vi "Channel Data to FP Cluster.vi"(0 "CS++DCPwrChannelData in":refnum<class "CS++DCPwrChannelData.lvclass">, 5 "Channel Index":i32, 11 "Error In":errorcluster) -> (2 "Maximum Limits":T2 {"Max Voltage Level" format="%^.3g"; "Max Current Limit" format="%^.3g"}, 3 "Range":cluster{"Range Type":i32, "Range":dbl}={"Range Type"=1, "Range"=0.0} {"Range" format="%^.3g"; "Range Type" items=["Voltage"=1, "Current"=0]}, 4 "CS++DCPwrChannelData out":refnum<class "CS++DCPwrChannelData.lvclass">, 6 "Output Enable":bool caption="Channel Enabled", 8 "Output State":i32(ring) items=["Constant Voltage"=0, "Constant Current"=1, "Unregulated"=4, "Over Voltage"=2, "Over Current"=3], 10 "Current":T1 {"Behavior" items=["Regulate", "Trip"]; "Current Limit" format="%^.3g"}, 13 "Trigger":T4 {"Triggered I-Limit" format="%^.6g"; "Triggered U-Level" format="%^.6g"; "Trigger Source" items=["Immediate", "External", "Software", "TTL0", "TTL1", "TTL2", "TTL3", "TTL4", "TTL5", "TTL6", "TTL7", "ECL0", "ECL1", "PXI Star", "RTSI 0", "RTSI 1", "RTSI 2", "RTSI 3", "RTSI 4", "RTSI 5", "RTSI 6"]}, 14 "OVP":T3 {"OVP Limit" format="%^.3g"}, 15 "Error Out":errorcluster)   [LabVIEW 2015, in "CS++DCPwrGui.lvlib" / "CS++DCPwrChannelData.lvclass"]
doc: "Return channel data in cluster ."
uses:
  CS++DCPwrChannelData/CS++DCPwrChannelData.lvclass
  CS++DCPwrChannelData/CS++DCPwrChannelData.lvclass/CS++DCPwrChannelData.ctl
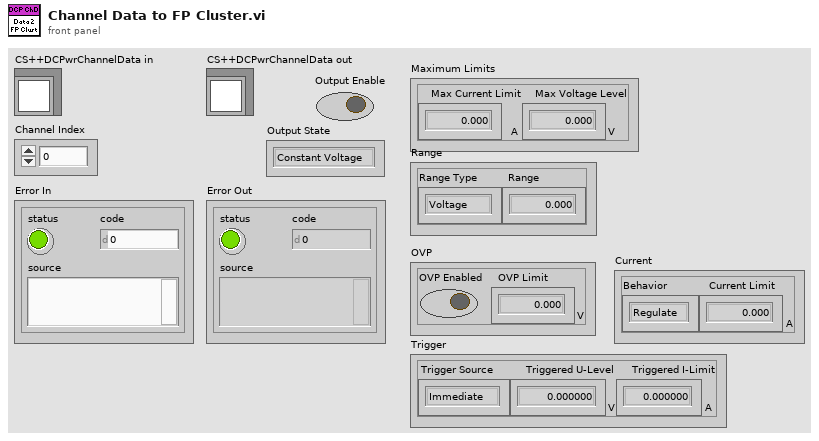
[diagram p1: front panel]
types:
  T1 = cluster{"Behavior":i32, "Current Limit":dbl[unit]}
  T2 = cluster{"Max Current Limit":dbl[unit], "Max Voltage Level":dbl[unit]}
  T3 = cluster{"OVP Enabled":bool, "OVP Limit":dbl[unit]}
  T4 = cluster{"Trigger Source":i32, "Triggered U-Level":dbl[unit], "Triggered I-Limit":dbl[unit]}
  T5 = cluster{"max current limit":dbl[unit], "max voltage level":dbl[unit]}
  T6 = cluster{"range type (Voltage)":i32, "range (0.0)":dbl}
  T7 = cluster{"behavior (regulate)":i32, "limit (0.0 Amps)":dbl[unit]}
  T8 = cluster{"enabled (true)":bool, "limit (0.0 Volts)":dbl[unit]}
  T9 = cluster{"source (Immediate)":i32, "triggered level (0.0 Volts)":dbl[unit], "triggered limit (0.0 Amps)":dbl[unit]}
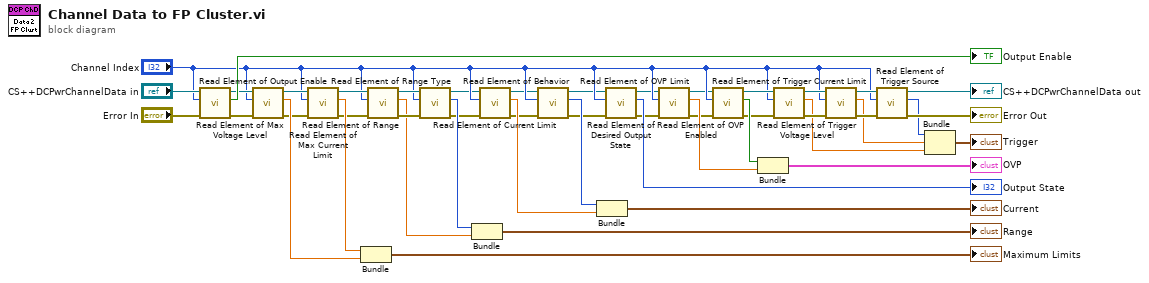
[diagram p0: block diagram]
diagram:
  n1 = call "Read Element of Output Enable.vi"("error in (no error)"="Error In", "index"="Channel Index", "CS++DCPwrChannelData in"="CS++DCPwrChannelData in") -> ("error out"=w41:errorcluster, "enabled (true)"=→"Output Enable":bool, "CS++DCPwrChannelData out"=w42:refnum<class "CS++DCPwrChannelData.lvclass">)  [unwired: 6 in]
  n2 = call "Read Element of Max Voltage Level.vi"("error in (no error)"=w41, "index"="Channel Index", "CS++DCPwrChannelData in"=w42) -> ("error out"=w39:errorcluster, "max voltage level"=w40:dbl[unit], "CS++DCPwrChannelData out"=w38:refnum<class "CS++DCPwrChannelData.lvclass">)  [unwired: 6 in]
  n3 = call "Read Element of Max Current Limit.vi"("error in (no error)"=w39, "index"="Channel Index", "CS++DCPwrChannelData in"=w38) -> ("error out"=w35:errorcluster, "max current limit"=w44:dbl[unit], "CS++DCPwrChannelData out"=w37:refnum<class "CS++DCPwrChannelData.lvclass">)  [unwired: 6 in]
  n4 = Bundle("max current limit"=w44, "max voltage level"=w40) -> (→"Maximum Limits":T5)  [unwired: 1 in]
  n5 = call "Read Element of Range.vi"("error in (no error)"=w35, "index"="Channel Index", "CS++DCPwrChannelData in"=w37) -> ("error out"=w34:errorcluster, "range (0.0)"=w32:dbl, "CS++DCPwrChannelData out"=w36:refnum<class "CS++DCPwrChannelData.lvclass">)  [unwired: 6 in]
  n6 = call "Read Element of Range Type.vi"("error in (no error)"=w34, "index"="Channel Index", "CS++DCPwrChannelData in"=w36) -> ("error out"=w8:errorcluster, "range type (Voltage)"=w33:i32, "CS++DCPwrChannelData out"=w7:refnum<class "CS++DCPwrChannelData.lvclass">)  [unwired: 6 in]
  n7 = Bundle("range type (Voltage)"=w33, "range (0.0)"=w32) -> (→"Range":T6)  [unwired: 1 in]
  n8 = call "Read Element of Current Limit.vi"("error in (no error)"=w8, "index"="Channel Index", "CS++DCPwrChannelData in"=w7) -> ("error out"=w5:errorcluster, "limit (0.0 Amps)"=w11:dbl[unit], "CS++DCPwrChannelData out"=w6:refnum<class "CS++DCPwrChannelData.lvclass">)  [unwired: 6 in]
  n9 = call "Read Element of Behavior.vi"("error in (no error)"=w5, "index"="Channel Index", "CS++DCPwrChannelData in"=w6) -> ("error out"=w3:errorcluster, "behavior (regulate)"=w10:i32, "CS++DCPwrChannelData out"=w4:refnum<class "CS++DCPwrChannelData.lvclass">)  [unwired: 6 in]
  n10 = Bundle("behavior (regulate)"=w10, "limit (0.0 Amps)"=w11) -> (→"Current":T7)  [unwired: 1 in]
  n11 = call "Read Element of Desired Output State.vi"("error in (no error)"=w3, "index"="Channel Index", "CS++DCPwrChannelData in"=w4) -> ("error out"=w2:errorcluster, "output state (Constant Voltage)"=→"Output State":i32, "CS++DCPwrChannelData out"=w1:refnum<class "CS++DCPwrChannelData.lvclass">)  [unwired: 6 in]
  n12 = call "Read Element of OVP Limit.vi"("error in (no error)"=w2, "index"="Channel Index", "CS++DCPwrChannelData in"=w1) -> ("error out"=w14:errorcluster, "limit (0.0 Volts)"=w30:dbl[unit], "CS++DCPwrChannelData out"=w15:refnum<class "CS++DCPwrChannelData.lvclass">)  [unwired: 6 in]
  n13 = call "Read Element of OVP Enabled.vi"("error in (no error)"=w14, "index"="Channel Index", "CS++DCPwrChannelData in"=w15) -> ("error out"=w27:errorcluster, "enabled (true)"=w31:bool, "CS++DCPwrChannelData out"=w28:refnum<class "CS++DCPwrChannelData.lvclass">)  [unwired: 6 in]
  n14 = Bundle("enabled (true)"=w31, "limit (0.0 Volts)"=w30) -> (→"OVP":T8)  [unwired: 1 in]
  n15 = call "Read Element of Trigger Current Limit.vi"("error in (no error)"=w27, "index"="Channel Index", "CS++DCPwrChannelData in"=w28) -> ("error out"=w23:errorcluster, "triggered limit (0.0 Amps)"=w17:dbl[unit], "CS++DCPwrChannelData out"=w26:refnum<class "CS++DCPwrChannelData.lvclass">)  [unwired: 6 in]
  n16 = call "Read Element of Trigger Voltage Level.vi"("error in (no error)"=w23, "index"="Channel Index", "CS++DCPwrChannelData in"=w26) -> ("error out"=w24:errorcluster, "triggered level (0.0 Volts)"=w18:dbl[unit], "CS++DCPwrChannelData out"=w25:refnum<class "CS++DCPwrChannelData.lvclass">)  [unwired: 6 in]
  n17 = call "Read Element of Trigger Source.vi"("error in (no error)"=w24, "index"="Channel Index", "CS++DCPwrChannelData in"=w25) -> ("error out"=→"Error Out":errorcluster, "source (Immediate)"=w19:i32, "CS++DCPwrChannelData out"=→"CS++DCPwrChannelData out":refnum<class "CS++DCPwrChannelData.lvclass">)  [unwired: 6 in]
  n18 = Bundle("source (Immediate)"=w19, "triggered level (0.0 Volts)"=w18, "triggered limit (0.0 Amps)"=w17) -> (→"Trigger":T9)  [unwired: 1 in]
